vi "Analyse error.vi"(8 "error in (no error)":errorcluster, 11 "IErrorHandler in":refnum<class "ErrorHandler MsgPack.lvclass">) -> (0 "error out":errorcluster, 3 "IErrorHandler out":refnum<class "ErrorHandler MsgPack.lvclass">)   [LabVIEW 2020, in "wamplv.lvlib" / "ErrorHandler MsgPack.lvclass"]
uses:
  ErrorHandler MsgPack.lvclass
  ErrorHandler MsgPack.lvclass/ErrorHandler MsgPack.ctl
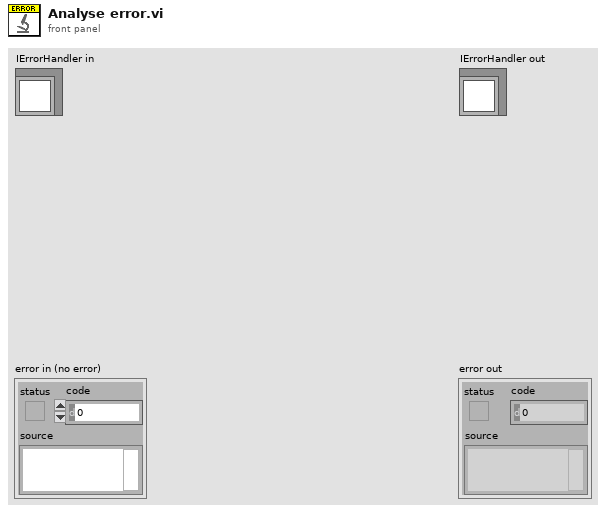
[diagram p1: front panel]
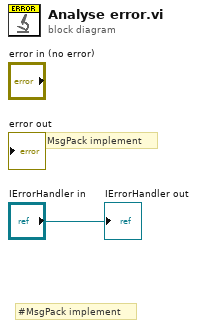
[diagram p0: block diagram]
diagram:
  # "#MsgPack implement"
  # "#MsgPack implement"
  "IErrorHandler out" <- "IErrorHandler in"
